vi "SetChannels.vi"(8 "error in (no error)":errorcluster, 10 "Channels":T1, 11 "NiPxi6733 in":refnum<class "NiPxi6733.lvclass">) -> (0 "error out":errorcluster, 3 "NiPxi6733 out":refnum<class "NiPxi6733.lvclass">)   [LabVIEW 2014, in "FgenPlugins.lvlib" / "NiPxi6733.lvclass"]
uses:
  NiPxi6733.lvclass
  TypeDefs/Channels.ctl
  TypeDefs/Channel.ctl
  FgenPluginBaseClass/FgenPluginsBase.lvclass/FgenPluginsBase.ctl
  FgenPluginBaseClass/Accessors/Read Channels.vi
  FgenPluginBaseClass/FgenPluginsBase.lvclass
  <resource>/objmgr/daqmx.rc
  FgenPlugins.lvlib
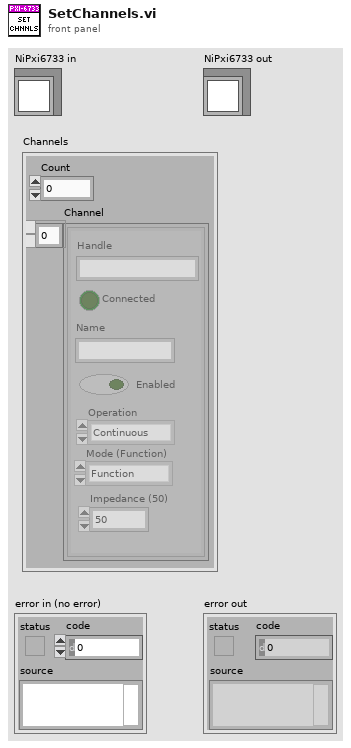
[diagram p1: front panel]
types:
  T1 = typedef "FgenPlugins.lvlib/Channels.ctl" = cluster{"Count":u16, "Channel":T2[]}
  T2 = typedef "FgenPlugins.lvlib/Channel.ctl" = cluster{"Name":string, "Enabled":bool, "Operation":enum16{"Continuous", "Burst"}, "Impedance (50)":dbl, "Handle":string, "Connected":bool, "Mode (Function)":enum16{"Function", "Arbitrary", "Sequence"}}
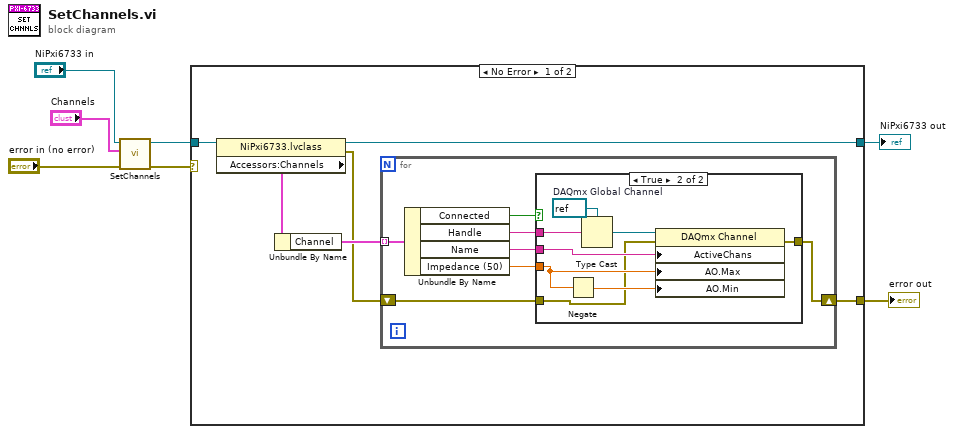
[diagram p0: block diagram]
diagram:
  n1 = call-parent "SetChannels.vi"("error in (no error)"="error in (no error)", "Channels"="Channels", "FgenPluginsBase in"="NiPxi6733 in") -> ("error out"=w4:errorcluster, "FgenPluginsBase out"=w3:refnum<class "NiPxi6733.lvclass">)  [unwired: 7 in]
  n2 = case shown="No Error" w4 {
    selector: w4 -> [_ w31]
    tunnel: w3 -> [w13 w30]
    tunnel: [w9 w31] -> w2
    tunnel: [w8 w30] -> w1
    frame No Error {
      n3 = property class="NiPxi6733.lvclass"(reference=w13) -> (reference out=w8:refnum<class "NiPxi6733.lvclass">, error out=w10:errorcluster, "Accessors:Channels"=w12:cluster{"Count":u16, "Channel":T2[]})  [unwired: 1 in]
      n4 = Unbundle By Name(w12) -> ("Channel"=w11:T2[])
      n5 = for {
        tunnel: w11 -> [w20] mode=indexing
        shift-right: [w14] -> w9
        shift-left: w10 -> [w15]
        n6 = Unbundle By Name(w20) -> ("Connected"=w19:bool, "Handle"=w18:string, "Name"=w17:string, "Impedance (50)"=w16:dbl)
        n7 = case shown="True" w19 {
          tunnel: w18 -> [_ w28]
          tunnel: w17 -> [_ w26]
          tunnel: w16 -> [_ w25]
          tunnel: w15 -> [w21 w23]
          tunnel: [w21 w22] -> w14
          frame False {
          }
          frame True {
            w29 = refnum<k21> refnum  # DAQmx Global Channel
            n8 = Negate(x=w25) -> (-x=w24:dbl)
            n9 = Type Cast(type=w29, x=w28) -> (*(type *) &x=w27:refnum<k21>)
            n10 = property class="DAQmx Channel"(reference=w27, error in=w23, "ActiveChans"=w26, "AO.Max"=w25, "AO.Min"=w24) -> (error out=w22:errorcluster)  [unwired: 1 out]
          }
        }
      }
    }
    frame Error {
    }
  }
  "error out" <- w2
  "NiPxi6733 out" <- w1
